vi "BuildLibraryImage.vi"(2 "Array":bool[](array[boolean]), 3 "Draw Area Size":T1, 4 "Books":string[](array[string])) -> (0 "Locations":T2(array[cluster]), 1 "new picture out":picture)   [LabVIEW 2012]
uses:
  <vilib>/Utility/miscctls.llb/LVBoundsTypeDef.ctl
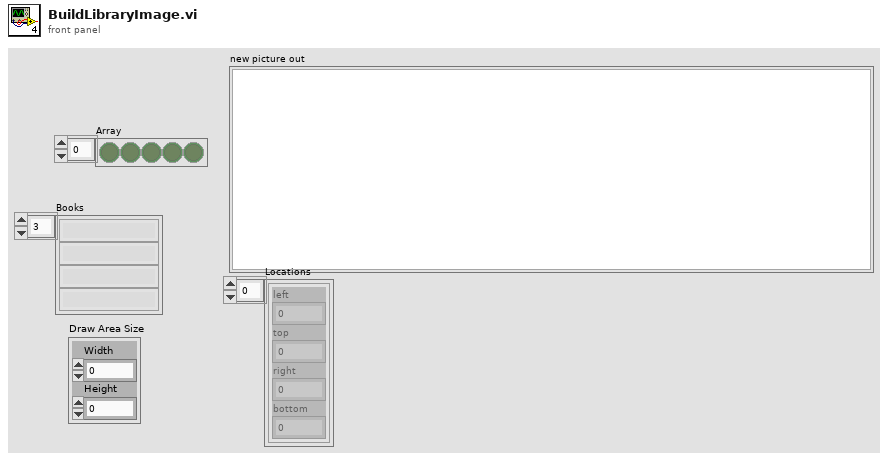
[diagram p1: front panel]
types:
  T1 = typedef "LVBoundsTypeDef.ctl" = cluster{"Width":u32, "Height":u32}
  T2 = cluster{"left":i32, "top":i32, "right":i32, "bottom":i32}[]
  T3 = typedef "QT_Image.ctl" = cluster{"Width":i32, "Height":i32, "Depth":i32, "data":u8[], "Compressed data":u8[], "Color table":u32[], "Duration":i32, "Options":i32, "Timestamp":i32, "ID":i32, "Reserved":i32, "Dialogs":u32}
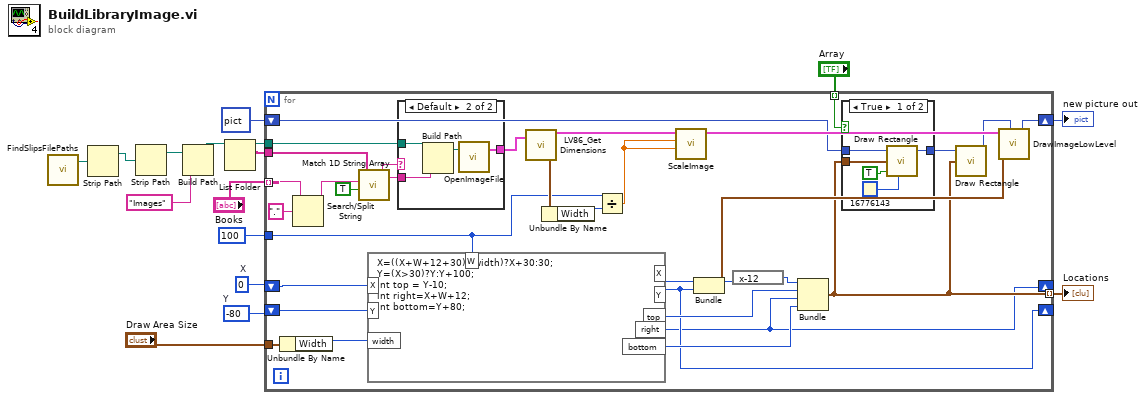
[diagram p0: block diagram]
diagram:
  w2 = -80  # Y
  w3 = 0  # X
  n1 = call "FindSlipsFilePaths.vi"() -> ("Slides"=w10:path)  [unwired: 2 in, 4 out]
  n2 = Strip Path(path=w10) -> (stripped path=w9:path)  [unwired: 1 out]
  n3 = Strip Path(path=w9) -> (stripped path=w8:path)  [unwired: 1 out]
  n4 = Build Path(base path=w8, name or relative path="Images") -> (appended path=w6:path)
  n5 = List Folder(path=w6) -> (path out=w12:path, filenames=w13:string[])  [unwired: 3 in, 2 out]
  n6 = for {
    tunnel: "Books" -> [w29] mode=indexing
    shift-right: [w33] -> w16
    shift-left: picture data[5B] ("new picture in") -> [w35]
    tunnel: w13 -> [w46]
    tunnel: w12 -> [w45]
    tunnel: 100 ("y") -> [w25]
    tunnel: "Array" -> [w32] mode=indexing
    tunnel: [w31] -> w4 mode=indexing
    shift-right: [w19] -> _
    shift-left: w3 -> [w26]
    shift-right: [w20] -> _
    shift-left: w2 -> [w24]
    tunnel: "Draw Area Size" -> [w18]
    n7 = Unbundle By Name(w18) -> ("Width"=w17:u32)
    n8 = Search/Split String(string=w29, search string/char (-)=".") -> (substring before match=w28:string)  [unwired: 1 in, 2 out]
    n9 = call <vilib>:"Match 1D String Array.vi"("Ignore Case? (false)"=TRUE, "Pattern"=w28, "Strings"=w46) -> ("Match"=w27:string)  [unwired: 1 in, 1 out]
    n10 = formula code="X=((X+W+12+30)<width)?X+30:30;\nY=(X>30)?Y:Y+100;\nint top = Y-10;\nint right=X+W+12;\nint bottom=Y+80;"("X"=w26, "Y"=w24, "W"=w25, "width"=w17) -> ("X"=w21:i32, "Y"=w20:i32, "top"=w22:i32, "right"=w19:i32, "bottom"=w23:i32)
    n11 = case shown="Default" w27 {
      tunnel: w27 -> [_ w50]
      tunnel: w45 -> [_ w49]
      tunnel: [_ w48] -> w40
      frame "" {
      }
      frame Default {
        n12 = Build Path(base path=w49, name or relative path=w50) -> (appended path=w51:path)
        n13 = call <userlib>:"OpenImageFile.vi"("selected path"=w51) -> ("Image Out"=w48:T3)  [unwired: 2 in]
      }
    }
    n14 = call <userlib>:"LV86_Get Dimensions.vi"("Image In"=w40) -> ("Dimensions"=w44:cluster{"Width":i32, "Height":i32}, "Image Out"=w42:T3)  [unwired: 1 in]
    n15 = Unbundle By Name(w44) -> ("Width"=w38:i32)
    n16 = Divide(x=w25, y=w38) -> (x/y=w41:dbl)
    n17 = call <userlib>:"ScaleImage.vi"("X scale"=w41, "Y scale"=w41, "Image in"=w42) -> ("Image Out"=w39:T3)  [unwired: 2 in]
    n18 = Bundle("X"=w21, "Y"=w20) -> (w43:cluster{"X":i32, "Y":i32})  [unwired: 1 in]
    n19 = expression code="x-12"(w21) -> (w37:i32)
    n20 = Bundle("X"=w37, w22, w19, w23) -> (w31:cluster{"X":i32, i32, i32, i32})  [unwired: 1 in]
    n21 = case shown="True" w32 {
      tunnel: [w56 w57] -> w36
      tunnel: w35 -> [w55 w57]
      tunnel: w31 -> [w54 _]
      frame True {
        n22 = call <vilib>:"Draw Rectangle.vi"("picture"=w55, "rect"=w54, "fill?(F)"=TRUE, "color(black)"=u32 16776143) -> ("new picture"=w56:picture)  [unwired: 5 in]
      }
      frame False {
      }
    }
    n23 = call <vilib>:"Draw Rectangle.vi"("picture"=w36, "rect"=w31) -> ("new picture"=w34:picture)  [unwired: 7 in]
    n24 = call <userlib>:"DrawImageLowLevel.vi"("Image"=w39, "Position"=w43, "picture in"=w34) -> ("new picture"=w33:picture)  [unwired: 2 in, 1 out]
  }
  "new picture out" <- w16
  "Locations" <- w4
